vi "Magnet_GUI.vi"(11 "GUI_cluster":T1={"Sub Panel"=refnum, "GUIdevice"="Bella_LP_Mode", "CtlRef"=refnum, "user event out"=refnum}) -> ()   [LabVIEW 2011]
uses:
  GUI_Template/GUI_master/tcp_new_data_event.ctl
  GUI_Template/GUI_master/tcp new data cluster.ctl
  Controls/GUI_cluster.ctl
  Controls/eventtypdef.ctl
panel:
  out "Boolean":bool
  in  "stop 2":refnum<vi>
  out "tcp data event":T2
  out "GUIdevice 1":string="Bella_LP_Mode"
  in  "stop":bool
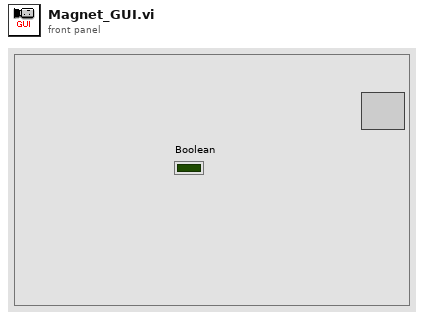
[diagram p1: front panel]
types:
  T1 = typedef "GUI_cluster.ctl" = cluster{"Sub Panel":refnum<vi>, "GUIdevice":string, "CtlRef":refnum<vi>, "user event out":refnum<user-event>}
  T2 = typedef "tcp_new_data_event.ctl" = refnum<user-event>
  T3 = typedef "eventtypdef.ctl" = cluster{"label":string, "Sub Panel":refnum<vi>, "CtlRef":refnum<vi>, "This VI":refnum<vi>}
  T4 = typedef "tcp new data cluster.ctl" = cluster{"EventEnum":enum16{"new data", "connection status update"}, "Device name":string}
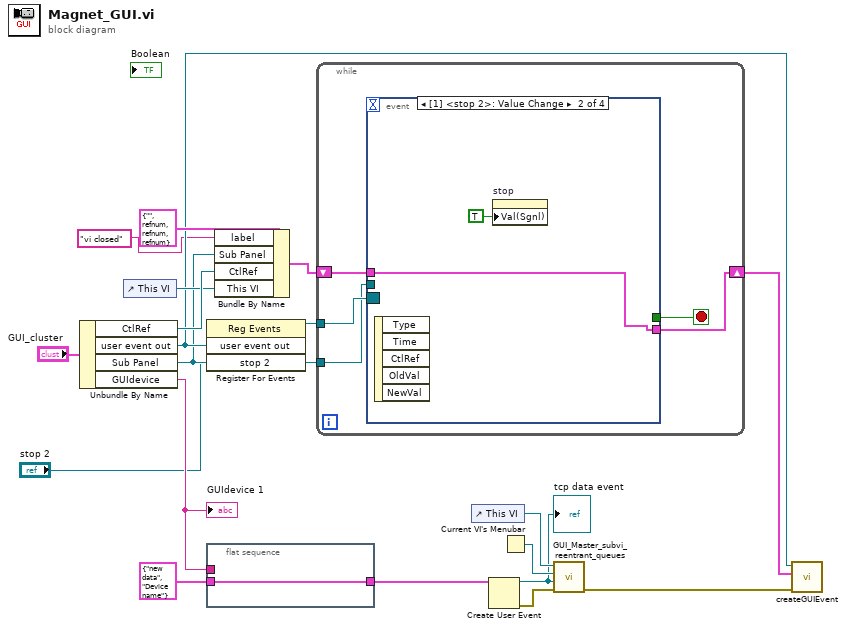
[diagram p0: block diagram]
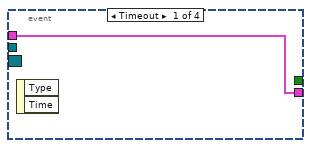
[diagram p2: hidden frame]
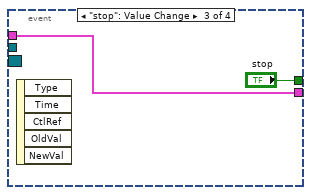
[diagram p3: hidden frame]
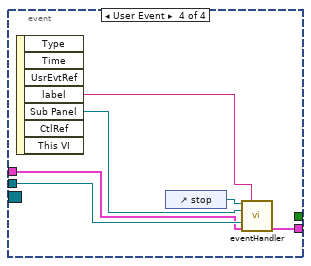
[diagram p4: hidden frame]
diagram:
  n1 = Unbundle By Name("GUI_cluster") -> ("CtlRef"=w11:refnum<vi>, "user event out"=w6:refnum<user-event>, "Sub Panel"=w4:refnum<vi>, "GUIdevice"=w9:string)
  "GUIdevice 1" <- w9
  n2 = control-ref of="This VI"() -> (w10:refnum<vi>)
  n3 = register-events(w6, "stop 2") -> (reference out=w5:refnum<event-registration>)  [unwired: 2 in, 1 out]
  n4 = flat-sequence {
    tunnel: T4 {"EventEnum"=enum."new data", "Device name"="Device name"} ("New Event") -> [w20]
    tunnel: [w20] -> w12
    tunnel: w9 -> [_]
    frame #0 {
    }
  }
  n5 = Bundle By Name(cluster=T3 {"label"="", "Sub Panel"=refnum, "CtlRef"=refnum, "This VI"=refnum} ("event data"), "label"="vi closed", "Sub Panel"=w4, "CtlRef"=w11, "This VI"=w10) -> (w7:T3)
  n6 = while {
    shift-right: [w23] -> w3
    shift-left: w7 -> [w24]
    tunnel: w5 -> [w22]
    tunnel: w4 -> [w21]
    stop <- w25 stop-if-true
    n7 = event shown="[1] <stop 2>: Value Change" {
      selector: w22 -> [_ _ _ _]
      dyn-events: _ -> [_ _ _ _]
      timeout: _ -> [_ _ _ _]
      tunnel: [_ _ "stop" _] -> w25
      tunnel: w24 -> [w26 w28 w29 w33]
      tunnel: [w26 w28 w29 w32] -> w23
      tunnel: w21 -> [_ _ _ w34]
      event Timeout {
        n8 = event-data() -> ()  [unwired: 1 in, 2 out]
      }
      event Value Change {
        n9 = event-data() -> ()  [unwired: 1 in, 5 out]
        n10 = property on="stop" class="Bool (strict)"("Val(Sgnl)"=TRUE ("Value (Signaling)")) -> ()  [unwired: 2 in, 2 out]
      }
      event "stop": Value Change {
        n11 = event-data() -> ()  [unwired: 1 in, 5 out]
      }
      event User Event {
        n12 = event-data() -> ("label"=w31:string, "Sub Panel"=w35:refnum<vi>)  [unwired: 1 in, 5 out]
        n13 = control-ref of="stop"() -> (w36:refnum<vi>)
        n14 = call "eventHandler.vi"("Boolean in"=w36, "label"=w31, "Sub Panel 2"=w35, "Sub Panel"=w34, "event data in"=w33) -> ("event data out"=w32:T3)  [unwired: 10 in]
      }
    }
  }
  n15 = control-ref of="This VI"() -> (w19:refnum<vi>)
  n16 = Create User Event(user event datatype=w12) -> (user event=w16:refnum<user-event>, error out=w17:errorcluster)  [unwired: 1 in]
  "tcp data event" <- w16
  n17 = Current VI's Menubar() -> (w18:refnum<k9>)
  n18 = call "GUI_Master_subvi_reentrant_queues.vi"("error in (no error)"=w17, "tcp data event"=w16, "Caller menu reference"=w18, "Caller VI ref"=w19) -> ("error out"=w8:errorcluster)  [unwired: 7 in]
  n19 = call "createGUIEvent.vi"("error in (no error)"=w8, "event data"=w3, "User Event in"=w6) -> ()  [unwired: 9 in]
